vi "Read width.vi"(8 "error in (no error)":errorcluster, 11 "Rectangle in":refnum<class "Rectangle.lvclass">) -> (0 "error out":errorcluster, 2 "width":dbl, 3 "Rectangle out":refnum<class "Rectangle.lvclass">)   [LabVIEW 2024, in "Rectangle.lvclass"]
uses:
  Rectangle.lvclass
  Rectangle.lvclass/Rectangle.ctl
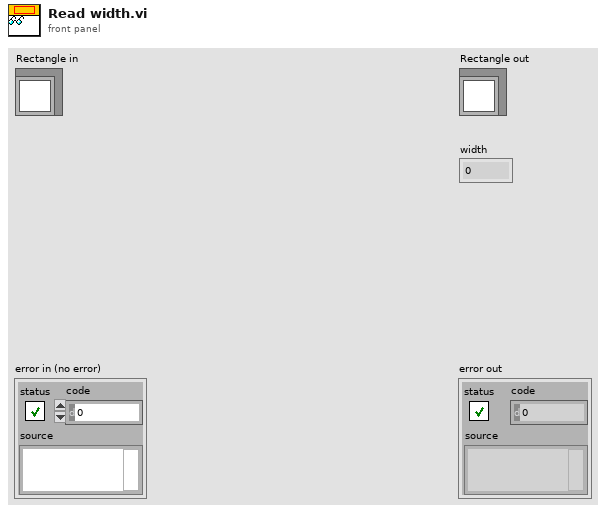
[diagram p1: front panel]
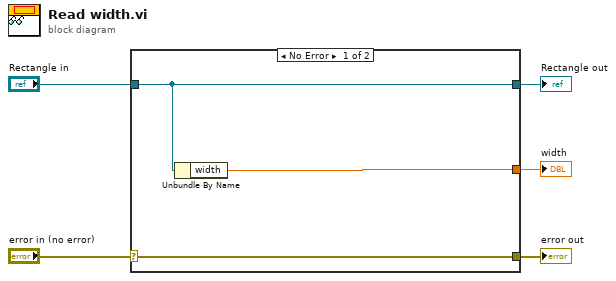
[diagram p0: block diagram]
diagram:
  n1 = case shown="No Error" "error in (no error)" {
    selector: "error in (no error)" -> [w8 w9]
    tunnel: [w8 w9] -> w4
    tunnel: [w7 w10] -> w2
    tunnel: "Rectangle in" -> [w7 w10]
    tunnel: [w6 _] -> w1
    frame No Error {
      n2 = Unbundle By Name(w7) -> ("width"=w6:dbl)
    }
    frame Error {
    }
  }
  "error out" <- w4
  "Rectangle out" <- w2
  "width" <- w1
